vi "Framework Configuration.Get Path.vi"(11 "Framework Configuration in":refnum<class "Framework Configuration.lvclass">) -> (2 "configuration path":path, 3 "Framework Configuration out":refnum<class "Framework Configuration.lvclass">)   [LabVIEW 2017, in "DSF.Engine.lvlib" / "Framework Configuration.lvclass"]
uses:
  Framework Configuration.lvclass
  Framework Configuration.lvclass/Framework Configuration.ctl
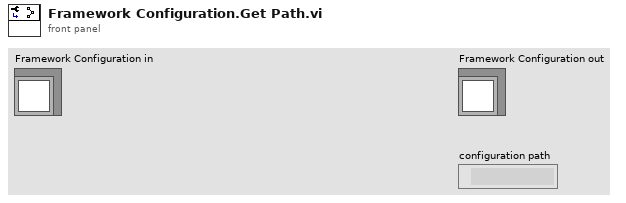
[diagram p1: front panel]
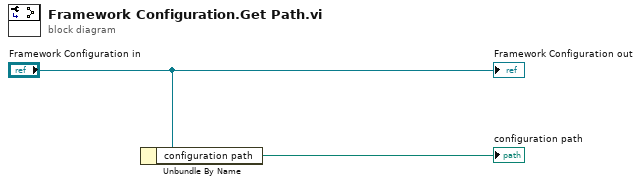
[diagram p0: block diagram]
diagram:
  n1 = Unbundle By Name("Framework Configuration in") -> ("configuration path"=→"configuration path":path)
  "Framework Configuration out" <- "Framework Configuration in"
